vi "Send Stop Notifier.vi"(8 "error in (no error)":errorcluster, 10 "Stop [T]":bool=TRUE, 11 "Transport in":refnum<class "Transport.lvclass">) -> (0 "error out":errorcluster, 3 "Transport out":refnum<class "Transport.lvclass">)   [LabVIEW 2019, in "Transport.lvclass"]
uses:
  Transport.lvclass
  Transport.lvclass/Transport.ctl
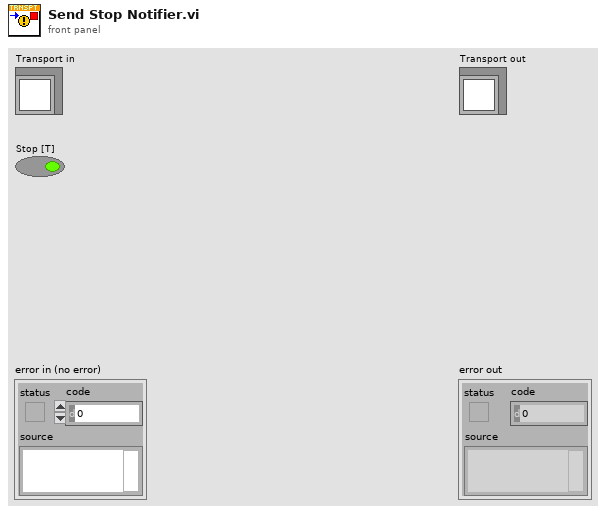
[diagram p1: front panel]
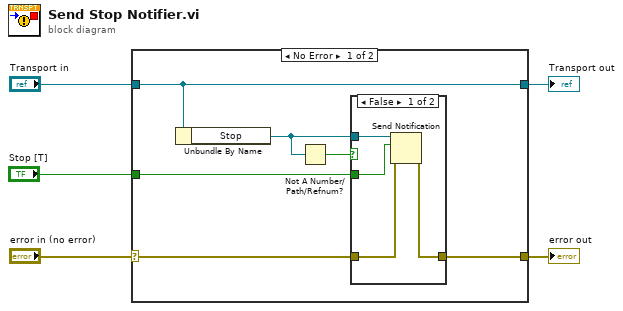
[diagram p0: block diagram]
diagram:
  n1 = case shown="No Error" "error in (no error)" {
    selector: "error in (no error)" -> [w11 w17]
    tunnel: [w10 w17] -> w4
    tunnel: [w6 w18] -> w2
    tunnel: "Transport in" -> [w6 w18]
    tunnel: "Stop [T]" -> [w9 _]
    frame No Error {
      n2 = Unbundle By Name(w6) -> ("Stop"=w7:refnum<notifier>)
      n3 = Not A Number/Path/Refnum?(number/path/refnum=w7) -> (NaN/Path/Refnum?=w8:bool)
      n4 = case shown="False" w8 {
        tunnel: w7 -> [w15 _]
        tunnel: w11 -> [w14 w16]
        tunnel: [w13 w16] -> w10
        tunnel: w9 -> [w12 _]
        frame False {
          n5 = Send Notification(notification=w12, notifier=w15, error in (no error)=w14) -> (error out=w13:errorcluster)  [unwired: 1 out]
        }
        frame True {
        }
      }
    }
    frame Error {
    }
  }
  "error out" <- w4
  "Transport out" <- w2
